vi "Convert.vi"(0 "Zaber":T1={"Serial port handle"="", "Axis"="", "Controller #"=0, "Min position"=0.0, "Max position"=0.0, "Min velocity"=0.0, "Max velocity"=0.0, "Firmware"="", "Device ID"=0, "Variable event"=refnum, "Variable ref"=refnum, "Resolution, usteps/step"=0, "Serial port semaphore"=refnum, "Joystick buttons"={"MinDir"=1, "MaxDir"=2, "MedSpeed"=5, "HighSpeed"=6}} {"Joystick buttons"."HighSpeed" min=1 max=25 step=1; "Joystick buttons"."MedSpeed" min=1 max=25 step=1; "Joystick buttons"."MaxDir" min=1 max=25 step=1; "Joystick buttons"."MinDir" min=1 max=25 step=1}, 1 "Position, mm":dbl, 2 "Velocity, mm/s":dbl, 3 "Accelaration, mm/s/s":dbl, 5 "error in":errorcluster, 6 "Position, usteps":i32, 8 "Velocity, counts":i32, 10 "Accelaration, counts":i32) -> (7 "Position, mm":dbl, 9 "Velocity, mm/s":dbl, 11 "Accelaration, mm/s/s":dbl, 14 "Zaber out":T1={"Serial port handle"="", "Axis"="", "Controller #"=0, "Min position"=0.0, "Max position"=0.0, "Min velocity"=0.0, "Max velocity"=0.0, "Firmware"="", "Device ID"=0, "Variable event"=refnum, "Variable ref"=refnum, "Resolution, usteps/step"=0, "Serial port semaphore"=refnum, "Joystick buttons"={"MinDir"=1, "MaxDir"=2, "MedSpeed"=5, "HighSpeed"=6}} {"Joystick buttons"."HighSpeed" min=1 max=25 step=1; "Joystick buttons"."MedSpeed" min=1 max=25 step=1; "Joystick buttons"."MaxDir" min=1 max=25 step=1; "Joystick buttons"."MinDir" min=1 max=25 step=1}, 15 "Position, usteps":i32, 16 "Velocity, counts":i32, 17 "Accelaration, counts":i32, 18 "Resolution, mm/ustep":dbl, 19 "error out":errorcluster)   [LabVIEW 2018]
uses:
  Zaber.ctl
  GenericDataEvent/GenericEvent.ctl
  ZaberVariables.ctl
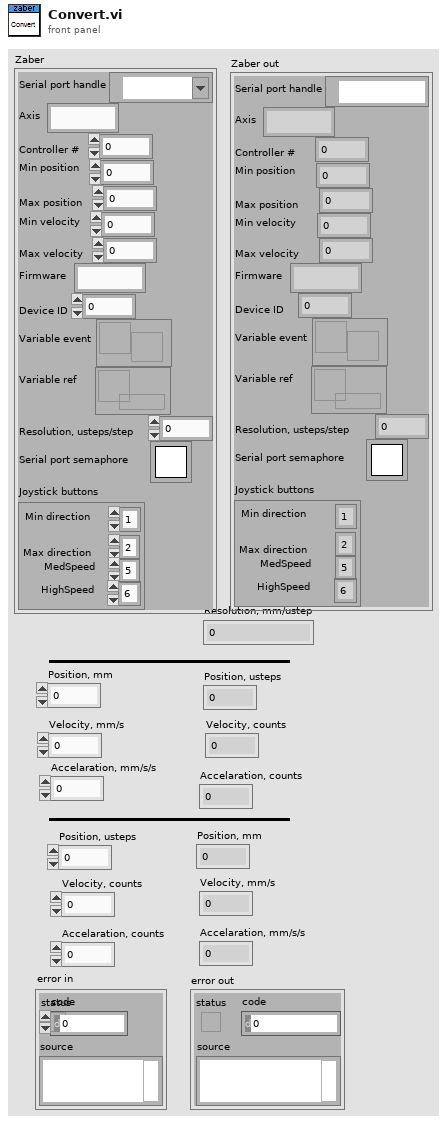
[diagram p1: front panel]
types:
  T1 = typedef "Zaber.ctl" = cluster{"Serial port handle":refnum<visa-resource-name>, "Axis":string, "Controller #":u8, "Min position":dbl, "Max position":dbl, "Min velocity":dbl, "Max velocity":dbl, "Firmware":string, "Device ID":i32, "Variable event":T2, "Variable ref":refnum<data-value>, "Resolution, usteps/step":i32, "Serial port semaphore":T3, "Joystick buttons":cluster{"MinDir":i32, "MaxDir":i32, "MedSpeed":i32, "HighSpeed":i32}}
  T2 = typedef "GenericEvent.ctl" = refnum<user-event>
  T3 = typedef "Semaphore RefNum" = refnum<k1>
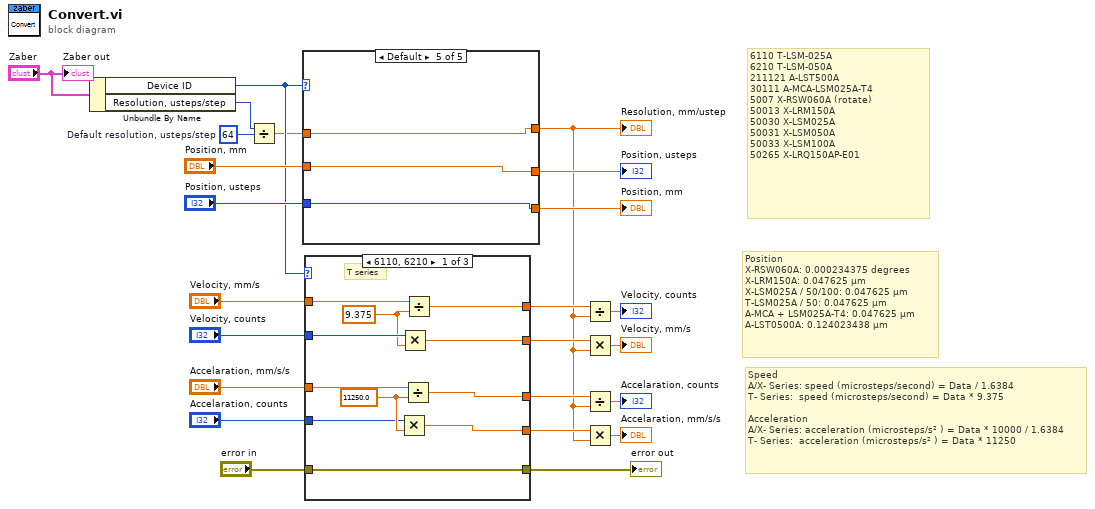
[diagram p0: block diagram]
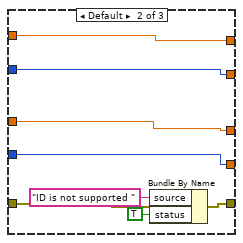
[diagram p2: hidden frame]
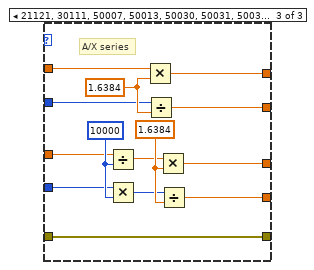
[diagram p3: hidden frame]
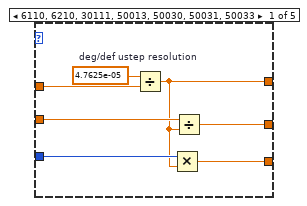
[diagram p4: hidden frame]
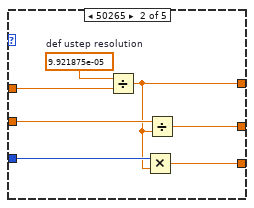
[diagram p5: hidden frame]
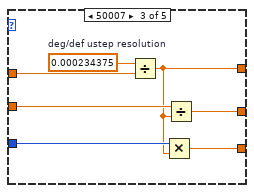
[diagram p6: hidden frame]
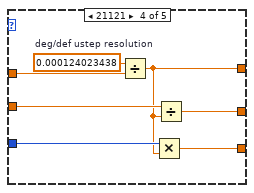
[diagram p7: hidden frame]
diagram:
  w14 = 64  # Default resolution, usteps/step
  # "6110 T-LSM-025A \n6210 T-LSM-050A\n211121 A-LST500A \n30111 A-MCA-LSM025A-T4\n5007 X-RSW060A (rotate)\n50013 X-LRM150A\n50030 X-LSM025A \n50031 X-LSM050A \n50033 X-LSM100A\n50265 X-LRQ150AP-E01"
  # "Speed\nA/X- Series: speed (microsteps/second) = Data / 1.6384\nT- Series:  speed (microsteps/second) = Data * 9.375\n\nAcceleration\nA/X- Series: acceleration (microsteps/s² ) = Data * 10000 / 1.6384\nT- Series:  acceleration (microsteps/s² ) = Data * 11250"
  # "Position\nX-RSW060A: 0.000234375 degrees\nX-LRM150A: 0.047625 µm\nX-LSM025A / 50/100: 0.047625 µm\nT-LSM025A / 50: 0.047625 µm\nA-MCA + LSM025A-T4: 0.047625 µm\nA-LST0500A: 0.124023438 µm"
  n1 = Unbundle By Name("Zaber") -> ("Device ID"=w20:i32, "Resolution, usteps/step"=w15:i32)
  n2 = Divide(x=w15, y=w14) -> (x/y=w13:dbl)
  n3 = case shown="Default" w20 {
    tunnel: "Position, usteps" -> [w31 w38 w41 w48 w53]
    tunnel: [w30 w37 w45 w52 w53] -> w22
    tunnel: "Position, mm" -> [w29 w36 w42 w49 w54]
    tunnel: [w28 w35 w39 w46 w54] -> w12
    tunnel: w13 -> [w26 w34 w43 w50 w55]
    tunnel: [w25 w33 w40 w47 w55] -> w4
    frame 6110, 6210, 30111, 50013, 50030, 50031, 50033 {
      w27 = 4.7625e-05  # deg/def ustep resolution
      n4 = Divide(x=w27, y=w26) -> (x/y=w25:dbl)
      n5 = Multiply(x=w31, y=w25) -> (x*y=w30:dbl)
      n6 = Divide(x=w29, y=w25) -> (x/y=w28:dbl)
    }
    frame 50265 {
      w32 = 9.921875e-05  # def ustep resolution
      n7 = Divide(x=w32, y=w34) -> (x/y=w33:dbl)
      n8 = Multiply(x=w38, y=w33) -> (x*y=w37:dbl)
      n9 = Divide(x=w36, y=w33) -> (x/y=w35:dbl)
    }
    frame 50007 {
      w44 = 0.000234375  # deg/def ustep resolution
      n10 = Divide(x=w44, y=w43) -> (x/y=w40:dbl)
      n11 = Multiply(x=w41, y=w40) -> (x*y=w45:dbl)
      n12 = Divide(x=w42, y=w40) -> (x/y=w39:dbl)
    }
    frame 21121 {
      w51 = 0.000124023438  # deg/def ustep resolution
      n13 = Divide(x=w51, y=w50) -> (x/y=w47:dbl)
      n14 = Multiply(x=w48, y=w47) -> (x*y=w52:dbl)
      n15 = Divide(x=w49, y=w47) -> (x/y=w46:dbl)
    }
    frame Default {
    }
  }
  "Resolution, mm/ustep" <- w4
  "Position, usteps" <- w12
  "Position, mm" <- w22
  n16 = case shown="6110, 6210" w20 {
    tunnel: "Velocity, mm/s" -> [w64 w74 w76]
    tunnel: "Velocity, counts" -> [w66 w73 w77]
    tunnel: "Accelaration, mm/s/s" -> [w59 w72 w81]
    tunnel: "Accelaration, counts" -> [w60 w71 w80]
    tunnel: [w65 w73 w88] -> w11
    tunnel: [w62 w74 w86] -> w7
    tunnel: [w58 w72 w79] -> w5
    tunnel: [w57 w71 w78] -> w9
    tunnel: "error in" -> [w56 w70 w75]
    tunnel: [w56 w68 w75] -> w1
    frame 6110, 6210 {
      w61 = 11250.0
      w63 = 9.375
      # "T series"
      n17 = Multiply(x=w60, y=w61) -> (x*y=w57:dbl)
      n18 = Multiply(x=w66, y=w63) -> (x*y=w65:dbl)
      n19 = Divide(x=w59, y=w61) -> (x/y=w58:dbl)
      n20 = Divide(x=w64, y=w63) -> (x/y=w62:dbl)
    }
    frame Default {
      n21 = Bundle By Name(cluster=w70, "source"="ID is not supported ", "status"=TRUE) -> (w68:errorcluster)
    }
    frame 21121, 30111, 50007, 50013, 50030, 50031, 50033, 50265 {
      w85 = 1.6384
      w83 = 10000 ("y")
      w87 = 1.6384
      # "A/X series"
      n22 = Divide(x=w81, y=w83) -> (x/y=w84:dbl)
      n23 = Multiply(x=w80, y=w83) -> (x*y=w82:i32)
      n24 = Multiply(x=w76, y=w87) -> (x*y=w86:dbl)
      n25 = Divide(x=w77, y=w87) -> (x/y=w88:dbl)
      n26 = Multiply(x=w84, y=w85) -> (x*y=w79:dbl)
      n27 = Divide(x=w82, y=w85) -> (x/y=w78:dbl)
    }
  }
  "error out" <- w1
  n28 = Divide(x=w7, y=w4) -> (x/y=→"Velocity, counts":dbl)
  n29 = Multiply(x=w11, y=w4) -> (x*y=→"Velocity, mm/s":dbl)
  n30 = Divide(x=w5, y=w4) -> (x/y=→"Accelaration, counts":dbl)
  n31 = Multiply(x=w9, y=w4) -> (x*y=→"Accelaration, mm/s/s":dbl)
  "Zaber out" <- "Zaber"
